vi "GatherJsonDataFromAPI.vi"() -> ()   [LabVIEW 2017]
uses:
  <vilib>/addons/_JKI.lib/REST Client/classes/REST Client/HTTP Header.ctl
  <vilib>/addons/_JKI.lib/REST Client/classes/REST Client/REST Client.lvclass
panel:
  out "Status String":string
  out "Response body":string
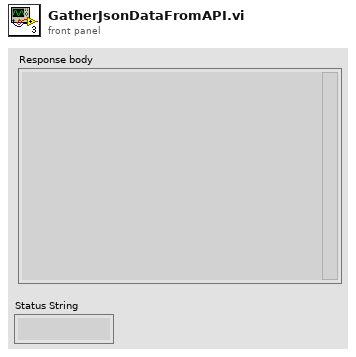
[diagram p1: front panel]
types:
  T1 = typedef "REST Client.lvlib/REST Client.lvclass/HTTP Header.ctl" = cluster{"header":string, "value":string}
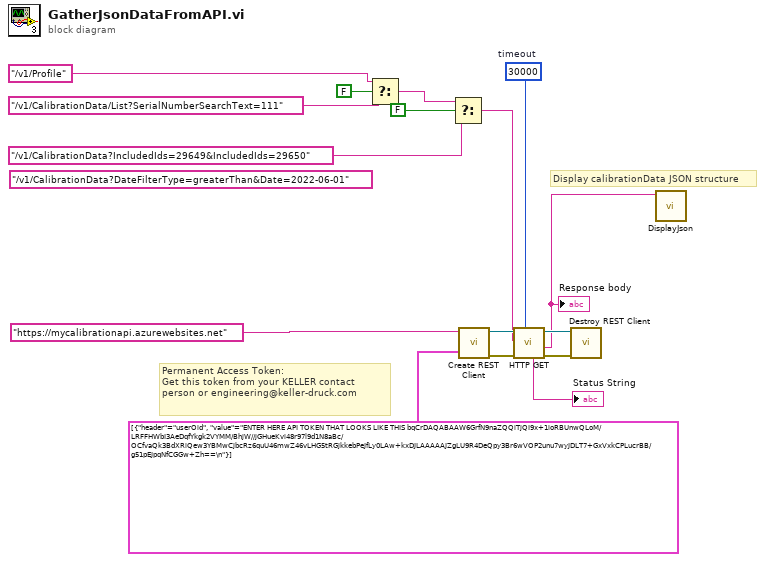
[diagram p0: block diagram]
diagram:
  w2 = 30000  # timeout
  (unwired) "/v1/CalibrationData?DateFilterType=greaterThan&Date=2022-06-01" ("Path")
  # "Display calibrationData JSON structure"
  # "Permanent Access Token:\nGet this token from your KELLER contact person or engineering@keller-druck.com"
  n1 = Select(t="/v1/Profile" ("Path"), s=FALSE, f="/v1/CalibrationData/List?SerialNumberSearchText=111" ("Path")) -> (s? t:f=w6:string)
  n2 = Select(t=w6, s=FALSE, f="/v1/CalibrationData?IncludedIds=29649&IncludedIds=29650" ("Path")) -> (s? t:f=w5:string)
  n3 = call <vilib>:"Create REST Client.vi"("Default Headers ([JSON])"=T1[] [{"header"="userOid", "value"="ENTER HERE API TOKEN THAT LOOKS LIKE THIS bqCrDAQABAAW6GrfN9naZQQiTjQI9x+1ioRBUnwQLoM/LRFFHWbI3AeDqfYkgk2VYMM/BhjW//jGHueKvi48r97l9d1N8aBc/OCfvaQk3BdXRiQew3YBMwCjbcRz6quU46mwZ46vLHG5tRGjkkebPeJfLy0LAw+kxDJLAAAAAJZgLU9R4DeQpy3Br6wVOP2unu7wyJDLT7+GxVxkCPLucrBB/g51pEJpqNfCGGw+Zh==\n"}], "Base URL"="https://mycalibrationapi.azurewebsites.net") -> ("error out"=w12:errorcluster, "REST Client out"=w15:refnum<class "REST Client.lvclass">)  [unwired: 8 in]
  n4 = call-dynamic "HTTP GET.vi"("timeout (0 = Use Default)"=w2, "error in (no error)"=w12, "Path"=w5, "REST Client in"=w15) -> ("error out"=w13:errorcluster, "Response body"=w3:string, "REST Client out"=w14:refnum<class "REST Client.lvclass">, "Status String"=→"Status String":string)  [unwired: 2 in, 2 out]
  "Response body" <- w3
  n5 = call-dynamic "Destroy REST Client.vi"("error in (no error)"=w13, "REST Client in"=w14) -> ()  [unwired: 9 in, 1 out]
  n6 = call "DisplayJson.vi"("JSON String In"=w3) -> ()  [unwired: 11 in]
